vi "float_to_real_3x1.vi"(10 "Float":dbl) -> (2 "REAL_3X1":string)   [LabVIEW 2018]
doc: "Format a float as an IC6 defined REAL_4X1 string."
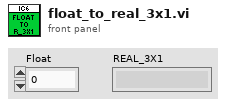
[diagram p1: front panel]
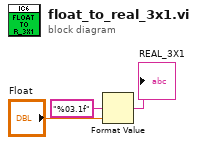
[diagram p0: block diagram]
diagram:
  n1 = Format Value(format string="%03.1f", value (0)="Float") -> (output string=→"REAL_3X1":string)  [unwired: 1 in]
